vi "Refresh Default Value.vi"(8 "error in (no error)":errorcluster, 10 "Label":T1 {"scheduleBuildUnit" items=["Millisecond", "Microsecond"]}, 11 "Param Ref in":T5 format="%.0x") -> (0 "error out":errorcluster, 3 "Param Ref out":T5 format="%.0x")   [LabVIEW 2017, in "Ballard Arinc-429 System Explorer.lvlib"]
uses:
  Ballard Arinc-429 System Explorer.lvlib
  <vilib>/NI Veristand/Custom Device API/Custom Device Item Ref.ctl
  Controls/Ballard_Label.ctl
  Controls/Ballard_Word.ctl
  Controls/ARINCParam.ctl
  Shared/Controls and Global/TransferType.ctl
  RT Driver/SubVIs/ReadWrite/Extract BCD Parameter.vi
  <vilib>/NI Veristand/Custom Device API/Get Item Property (Double).vi
  <vilib>/NI Veristand/Custom Device API/Get Item Property (I32).vi
  <vilib>/NI Veristand/Custom Device API/Get Item Property (Boolean).vi
  <vilib>/NI Veristand/Custom Device Tools/Custom Device Utility Library/NI VeriStand - Search for All Items by GUID.vi
  <vilib>/NI Veristand/Custom Device Tools/Custom Device Utility Library/NI VeriStand - Search for Item by GUID.vi
  Shared/Controls and Global/Global.vi
  Shared/Ballard Arinc-429 Shared.lvlib
  <vilib>/NI Veristand/Custom Device API/Custom Device API.lvlib
  <vilib>/NI Veristand/Custom Device Tools/Custom Device Utility Library/Custom Device Utility Library.lvlib
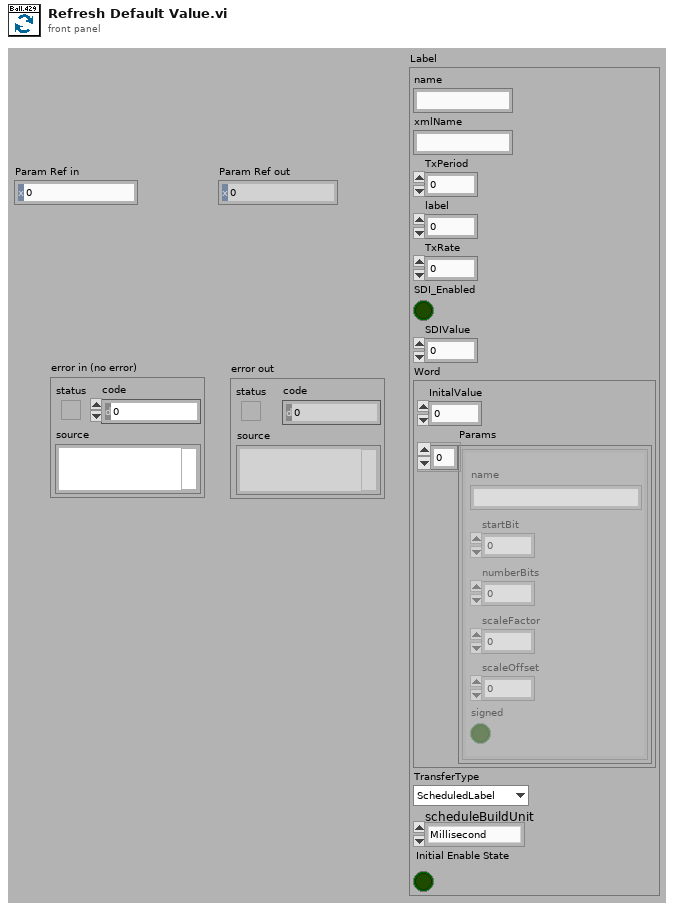
[diagram p1: front panel]
types:
  T1 = typedef "Ballard Arinc-429 System Explorer.lvlib/Ballard_Label.ctl" = cluster{"name":string, "xmlName":string, "TxPeriod":u32, "label":u32, "TxRate":dbl, "SDI_Enabled":bool, "SDIValue":u8, "Word":T2, "TransferType":T4, "scheduleBuildUnit":i32, "Initial Enable State":bool}
  T2 = typedef "Ballard Arinc-429 System Explorer.lvlib/Ballard_Word.ctl" = cluster{"InitalValue":u32, "Params":T3[]}
  T3 = typedef "Ballard Arinc-429 System Explorer.lvlib/ARINCParam.ctl" = cluster{"name":string, "startBit":i32, "numberBits":i32, "scaleFactor":dbl, "scaleOffset":dbl, "signed":bool}
  T4 = typedef "Ballard Arinc-429 Shared.lvlib/TransferType.ctl" = enum16{"ScheduledLabel", "Acyclic", "Block", "Strobe"}
  T5 = typedef "Custom Device API.lvlib/Custom Device Item Ref.ctl" = u64
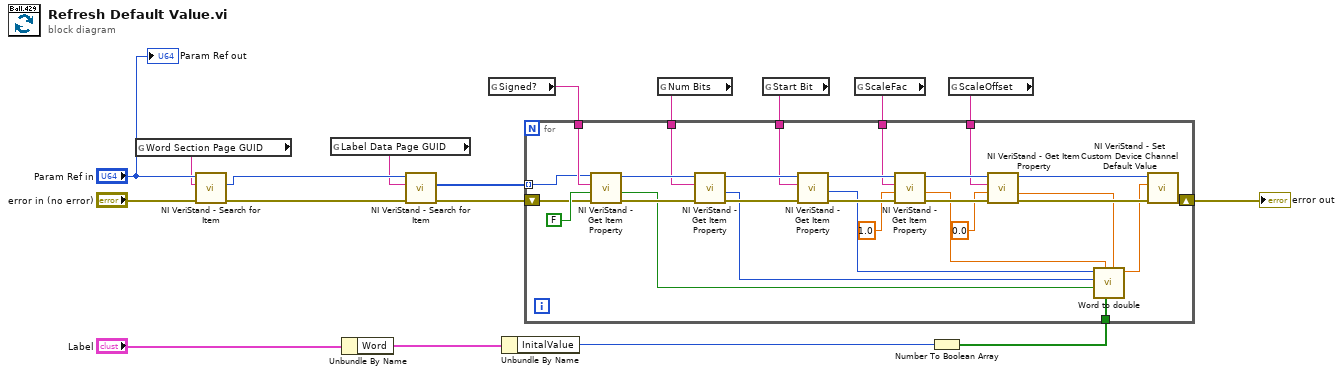
[diagram p0: block diagram]
diagram:
  n1 = global read "Global.vi" "Word Section Page GUID"() -> (w14:string)
  n2 = call-poly <vilib>:"NI VeriStand - Search for Item.vi"("error in"="error in (no error)", "Item GUID"=w14, "Section Ref in"="Param Ref in") -> ("error out"=w16:errorcluster, "Item Ref"=w13:T5)  [unwired: 5 in, 2 out]
  n3 = global read "Global.vi" "Label Data Page GUID"() -> (w6:string)
  n4 = Unbundle By Name("Label") -> ("Word"=w1:T2)
  n5 = call-poly <vilib>:"NI VeriStand - Search for Item.vi"("error in"=w16, "Item GUID"=w6, "Section Ref in"=w13) -> ("error out"=w5:errorcluster, "Item Refs"=w4:T5[])  [unwired: 5 in, 2 out]
  n6 = global read "Global.vi" "Signed?"() -> (w11:string)
  n7 = Unbundle By Name(w1) -> ("InitalValue"=w3:u32)
  n8 = global read "Global.vi" "Num Bits"() -> (w10:string)
  n9 = global read "Global.vi" "Start Bit"() -> (w9:string)
  n10 = global read "Global.vi" "ScaleFac"() -> (w8:string)
  n11 = Number To Boolean Array(number=w3) -> (Boolean array=w2:bool[])
  n12 = global read "Global.vi" "ScaleOffset"() -> (w7:string)
  n13 = for {
    tunnel: w2 -> [w19]
    tunnel: w11 -> [w46]
    tunnel: w10 -> [w42]
    tunnel: w9 -> [w39]
    tunnel: w8 -> [w34]
    tunnel: w7 -> [w31]
    shift-right: [w28] -> w18
    shift-left: w5 -> [w20]
    tunnel: w4 -> [w21] mode=indexing
    n14 = call-poly <vilib>:"NI VeriStand - Get Item Property.vi"("error in (no error)"=w20, "Default Value"=FALSE, "Property Name"=w46, "Item Ref in"=w21) -> ("error out"=w45:errorcluster, "Value"=w22:bool, "Item Ref out"=w44:T5)  [unwired: 4 in, 1 out]
    n15 = call-poly <vilib>:"NI VeriStand - Get Item Property.vi"("error in (no error)"=w45, "Property Name"=w42, "Item Ref in"=w44) -> ("error out"=w41:errorcluster, "Value"=w23:i32, "Item Ref out"=w40:T5)  [unwired: 5 in, 1 out]
    n16 = call-poly <vilib>:"NI VeriStand - Get Item Property.vi"("error in (no error)"=w41, "Property Name"=w39, "Item Ref in"=w40) -> ("error out"=w38:errorcluster, "Value"=w24:i32, "Item Ref out"=w37:T5)  [unwired: 5 in, 1 out]
    n17 = call-poly <vilib>:"NI VeriStand - Get Item Property.vi"("error in (no error)"=w38, "Default Value"=1.0 ("Scale Factor"), "Property Name"=w34, "Item Ref in"=w37) -> ("error out"=w35:errorcluster, "Value"=w25:dbl, "Item Ref out"=w36:T5)  [unwired: 4 in, 1 out]
    n18 = call-poly <vilib>:"NI VeriStand - Get Item Property.vi"("error in (no error)"=w35, "Default Value"=0.0 ("Scale Factor"), "Property Name"=w31, "Item Ref in"=w36) -> ("error out"=w30:errorcluster, "Value"=w26:dbl, "Item Ref out"=w29:T5)  [unwired: 4 in, 1 out]
    n19 = call "Word to double.vi"("ScaleOffset (0)"=w26, "Word"=w19, "ScaleFac (1)"=w25, "Signed? (F)"=w22, "Number of Bits"=w23, "Start Bit"=w24) -> ("Double"=w27:dbl)  [unwired: 5 in]
    n20 = call <vilib>:"NI VeriStand - Set Custom Device Channel Default Value.vi"("error in (no error)"=w30, "Default Value"=w27, "Channel Ref in"=w29) -> ("error out"=w28:errorcluster)  [unwired: 7 in, 1 out]
  }
  "error out" <- w18
  "Param Ref out" <- "Param Ref in"
